vi "Globals.vi"() -> ()   [LabVIEW 2014]
uses:
  TCP_IP/TCP_IP.lvclass
panel:
  in  "Return Data":string
  in  "Log History":string
  in  "Exit Measurement":bool
  in  "connection ID":refnum<k5>
  in  "TCP_IP":refnum<class "TCP_IP.lvclass">
  in  "Log":string
  in  "Restart Network":bool
  in  "Stop":bool
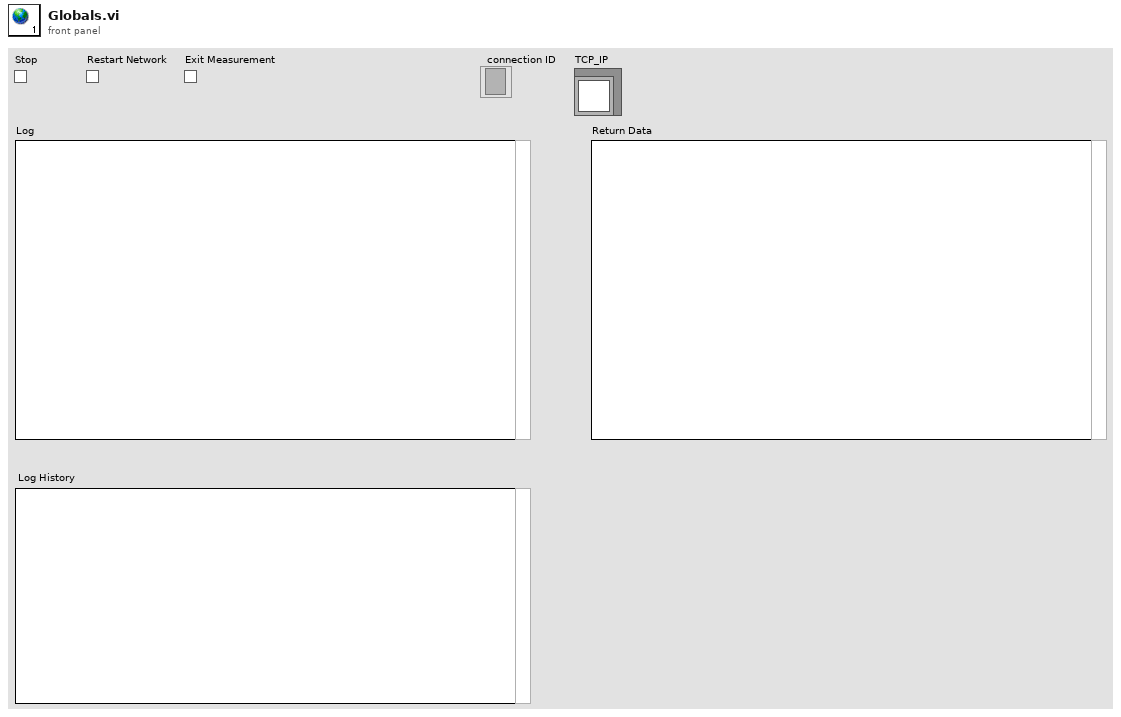
[diagram p1: front panel]
diagram:
